vi "Central Update.vi"(11 "ref in":refnum<k20>) -> (3 "ref out":refnum<k20>)   [LabVIEW 2019]
uses:
  RT Controls/Top Dome Status.ctl
  RT Controls/FPGA State.ctl
  RT Controls/Main Box Status.ctl
  RT Controls/Rotation Status.ctl
  RT Controls/Last Rotation.ctl
  RT Controls/Homing State.ctl
  RT Controls/Main Box Config.ctl
  RT Controls/Main Box Control.ctl
  RT Controls/Main Box Buttons.ctl
  <vilib>/Utility/error.llb/Error Cluster From Error Code.vi
  <vilib>/rvi/errors/niLvFpgaAdjustHostInterfaceError.vi
  <vilib>/rvi/interface/nirviReadWriteControl/nirviReadWriteControl.xnode
  <vilib>/rvi/interface/Simulation/niFpgaSimulationCallBeginRW.vi
  NiFpgaLv.dll
panel:
  out "shutdown":bool
  out "FPGA State":T1
  out "mode":u8
  out "sub mode":u8
  out "cmd":i8
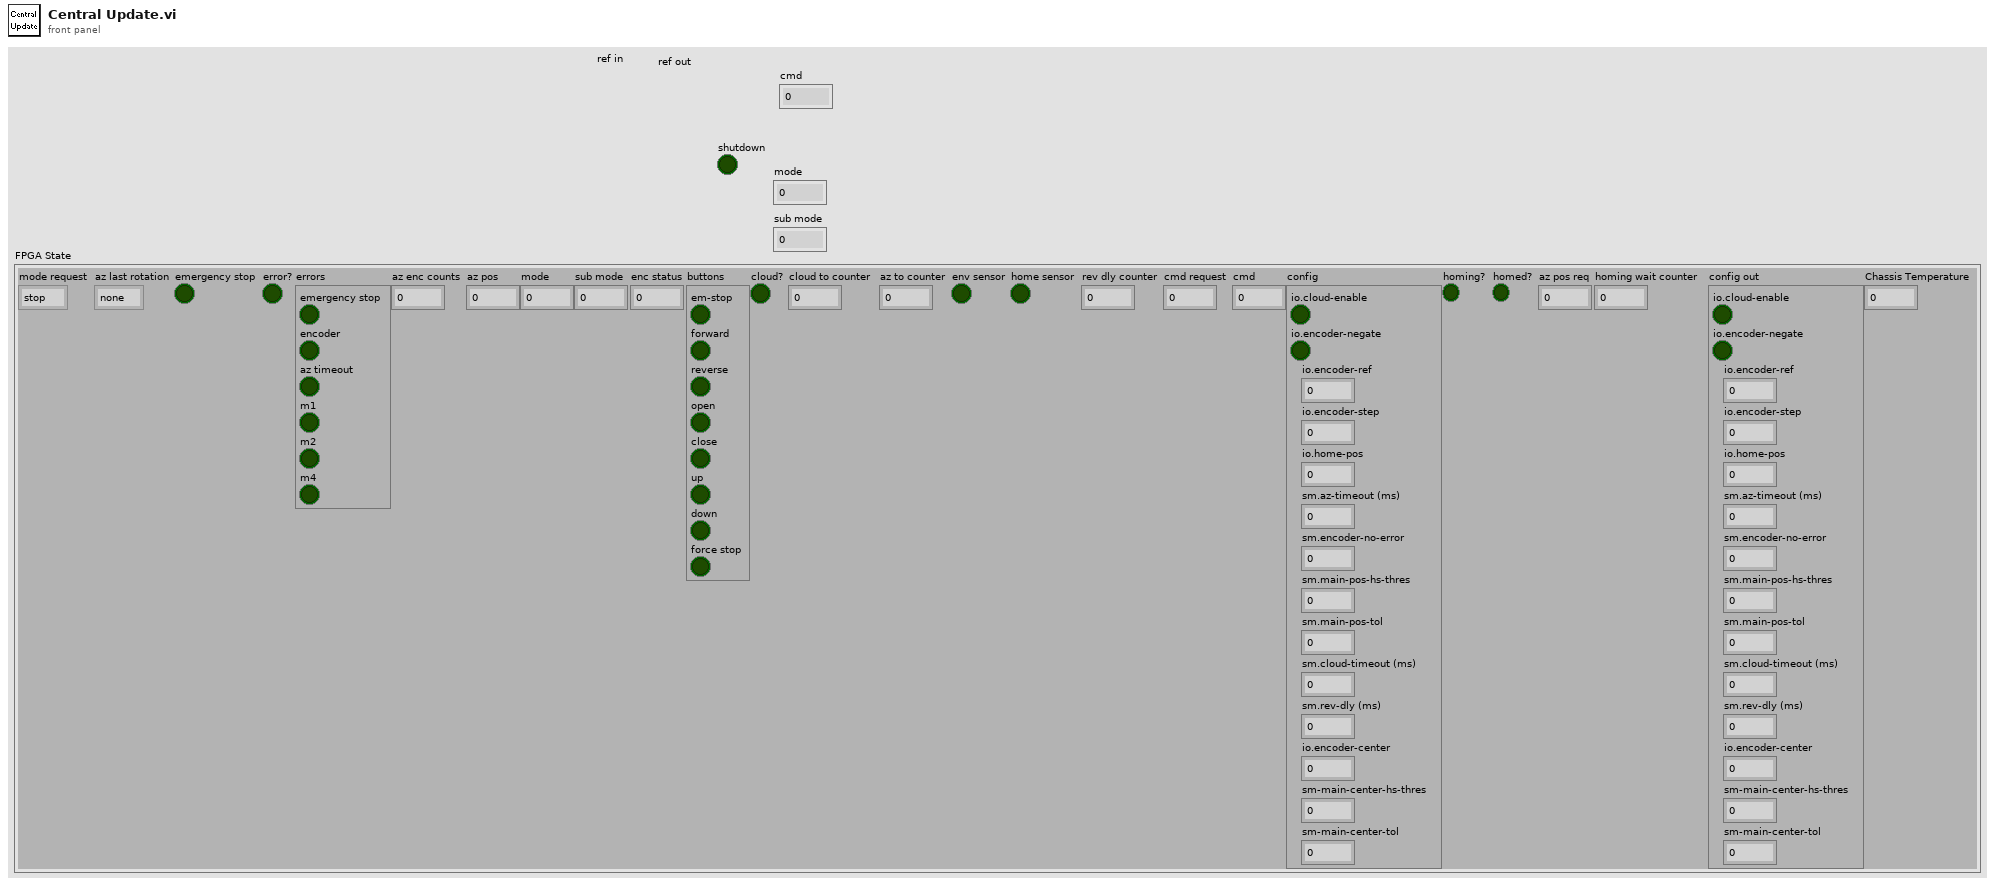
[diagram p1: front panel]
types:
  T1 = cluster{"mode request":enum16{"stop", "home", "position", "center"}, "az last rotation":enum16{"none", "forward", "reverse"}, "emergency stop":bool, "error?":bool, "errors":cluster{"emergency stop":bool, "encoder":bool, "az timeout":bool, "m1":bool, "m2":bool, "m4":bool}, "az enc counts":u64, "az pos":fxp<+/-,32,2>, "mode":u8, "sub mode":u8, "enc status":u16, "buttons":cluster{"em-stop":bool, "forward":bool, "reverse":bool, "open":bool, "close":bool, "up":bool, "down":bool, "force stop":bool}, "cloud?":bool, "cloud to counter":u32, "az to counter":u32, "env sensor":bool, "home sensor":bool, "rev dly counter":u32, "cmd request":i8, "cmd":i8, "config":cluster{"io.cloud-enable":bool, "io.encoder-negate":bool, "io.encoder-ref":u64, "io.encoder-step":u64, "io.home-pos":fxp<+/-,32,2>, "sm.az-timeout (ms)":u32, "sm.encoder-no-error":u16, "sm.main-pos-hs-thres":fxp<+/-,32,2>, "sm.main-pos-tol":fxp<+/-,32,2>, "sm.cloud-timeout (ms)":u32, "sm.rev-dly (ms)":u32, "io.encoder-center":u64, "sm-main-center-hs-thres":u64, "sm-main-center-tol":u64}, "homing?":bool, "homed?":bool, "az pos req":fxp<+/-,32,2>, "homing wait counter":u32, "config out":cluster{"io.cloud-enable":bool, "io.encoder-negate":bool, "io.encoder-ref":u64, "io.encoder-step":u64, "io.home-pos":fxp<+/-,32,2>, "sm.az-timeout (ms)":u32, "sm.encoder-no-error":u16, "sm.main-pos-hs-thres":fxp<+/-,32,2>, "sm.main-pos-tol":fxp<+/-,32,2>, "sm.cloud-timeout (ms)":u32, "sm.rev-dly (ms)":u32, "io.encoder-center":u64, "sm-main-center-hs-thres":u64, "sm-main-center-tol":u64}, "Chassis Temperature":i16}
  T2 = typedef "Homing State.ctl" = enum16{"Idle", "SlewFwd", "SlewRev", "SeekFwd", "SeekRev", "AtHome", "FwdWait", "RevWait"}
  T3 = typedef "Last Rotation.ctl" = enum16{"--", "RR", "RL"}
  T4 = typedef "Rotation Status.ctl" = enum16{"Stop", "Left", "Right", "Homing"}
  T5 = typedef "Top Dome Status.ctl" = cluster{"UpperDoorStatus":enum16{"Ajar", "Open", "Shut", "Error"}, "LowerDoorStatus":enum16{"Ajar", "Shut", "Open", "Error"}, "EM Button":bool, "WDTime":bool, "AutoShut":bool, "Rain":bool, "Interlock":bool, "UpperDoorEl":dbl, "LowerDoorEl":dbl, "UpperDoorEnc":u64, "LowerDoorEnc":u64}
  T6 = cluster{"emergency stop":bool, "encoder":bool, "az timeout":bool, "m1":bool, "m2":bool, "m4":bool}
  T7 = cluster{"em-stop":bool, "forward":bool, "reverse":bool, "open":bool, "close":bool, "up":bool, "down":bool, "force stop":bool}
  T8 = cluster{"io.cloud-enable":bool, "io.encoder-negate":bool, "io.encoder-ref":u64, "io.encoder-step":u64, "io.home-pos":fxp<+/-,32,2>, "sm.az-timeout (ms)":u32, "sm.encoder-no-error":u16, "sm.main-pos-hs-thres":fxp<+/-,32,2>, "sm.main-pos-tol":fxp<+/-,32,2>, "sm.cloud-timeout (ms)":u32, "sm.rev-dly (ms)":u32, "io.encoder-center":u64, "sm-main-center-hs-thres":u64, "sm-main-center-tol":u64}
  T9 = typedef "Main Box Config.ctl" = cluster{"WatchdogTim":i32, "DirRevDel":i32, "Coast":dbl, "HSThres":dbl, "EncCounts360":u64, "HomePos":dbl, "EncRefDeg":dbl, "EncRefCounts":u64, "Tol":dbl, "CloudEn":bool, "AutoShutEn":bool, "RainTim":i32, "AZTimeout":i32, "AZEncPol":enum16{"Positive", "Negative"}}
  T10 = typedef "Main Box Status.ctl" = cluster{"RotStatus":T4, "EMButton":bool, "TopComms":bool, "CurAZ":dbl, "At Home":bool, "LastRot":T3, "Cloud":bool, "CurAZEnc":u64, "LastAZ":dbl, "AutoShut":bool, "WDTime":bool, "HomeState":T2}
  T11 = typedef "Main Box Control.ctl" = cluster{"ForwardDome":bool, "ReverseDome":bool, "GotoHome":bool, "HighSpeed":bool}
  T12 = typedef "Main Box Buttons.ctl" = cluster{"EMStop":bool, "CloseMainDoor":bool, "OpenMainDoor":bool, "CloseLowerDoor":bool, "OpenLowerDoor":bool, "ForwardDome":bool, "ReverseDome":bool}
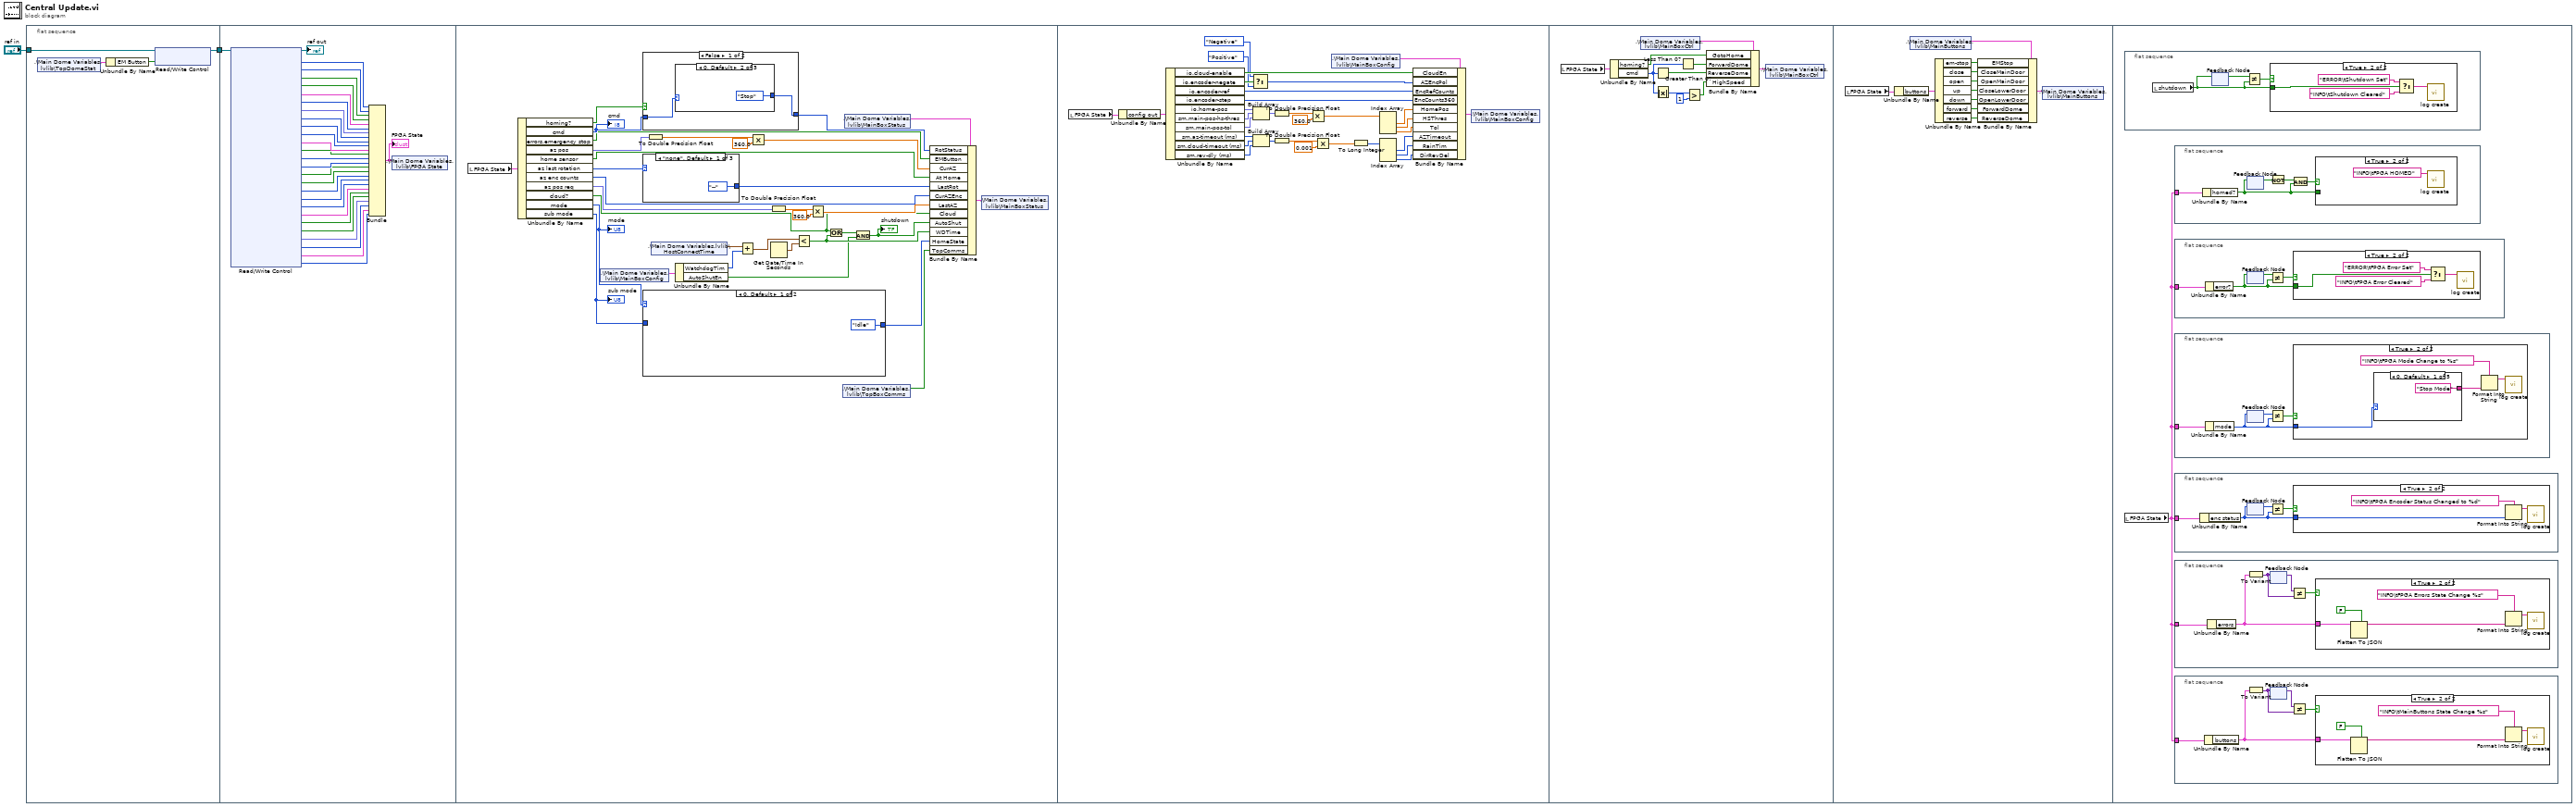
[diagram p0: block diagram]
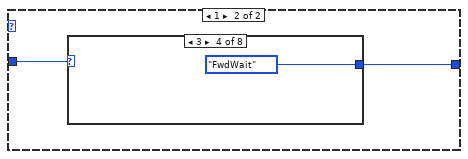
[diagram p2: hidden frame]
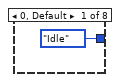
[diagram p3: hidden frame]
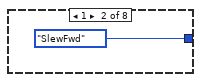
[diagram p4: hidden frame]
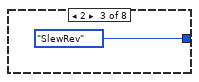
[diagram p5: hidden frame]
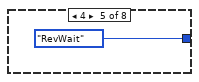
[diagram p6: hidden frame]
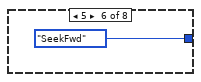
[diagram p7: hidden frame]
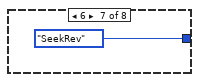
[diagram p8: hidden frame]
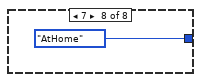
[diagram p9: hidden frame]
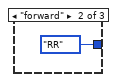
[diagram p10: hidden frame]
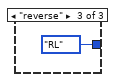
[diagram p11: hidden frame]
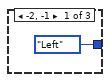
[diagram p12: hidden frame]
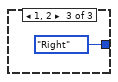
[diagram p13: hidden frame]
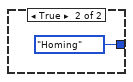
[diagram p14: hidden frame]
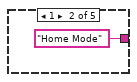
[diagram p20: hidden frame]
diagram:
  n1 = flat-sequence {
    tunnel: "ref in" -> [w6]
    tunnel: [w5] -> w2
    tunnel: w2 -> [w35]
    frame #0 {
      n2 = shared-variable ".\\Main Dome Variables.lvlib\\TopDomeStat"() -> (w4:T5)  [unwired: 1 in, 1 out]
      n3 = Unbundle By Name(w4) -> ("EM Button"=w3:bool)
      n4 = xnode "Read/Write Control"("FPGA VI Reference In"=w6, "emergency stop"=w3) -> ("FPGA VI Reference Out"=w5:refnum<k20>)  [unwired: 1 in, 1 out]
    }
    frame #1 {
      n5 = xnode "Read/Write Control"("FPGA VI Reference In"=w35) -> ("FPGA VI Reference Out"=→"ref out":refnum<k20>, "mode request"=w34:enum16{"stop", "home", "position", "center"}, "az last rotation"=w33:enum16{"none", "forward", "reverse"}, "emergency stop"=w32:bool, "error?"=w31:bool, "errors"=w30:T6, "az enc counts"=w29:u64, "az pos"=w28:fxp<+/-,32,2>, "mode"=w27:u8, "sub mode"=w26:u8, "enc status"=w25:u16, "buttons"=w24:T7, "cloud?"=w23:bool, "cloud to counter"=w22:u32, "az to counter"=w21:u32, "env sensor"=w20:bool, "home sensor"=w19:bool, "rev dly counter"=w18:u32, "cmd request"=w17:i8, "cmd"=w16:i8, "config"=w15:T8, "homing?"=w14:bool, "homed?"=w9:bool, "az pos req"=w13:fxp<+/-,32,2>, "homing wait counter"=w12:u32, "config out"=w11:T8, "Chassis Temperature"=w10:i16)  [unwired: 1 in, 1 out]
      n6 = Bundle("mode request"=w34, "az last rotation"=w33, "emergency stop"=w32, "error?"=w31, "errors"=w30, "az enc counts"=w29, "az pos"=w28, "mode"=w27, "sub mode"=w26, "enc status"=w25, "buttons"=w24, "cloud?"=w23, "cloud to counter"=w22, "az to counter"=w21, "env sensor"=w20, "home sensor"=w19, "rev dly counter"=w18, "cmd request"=w17, "cmd"=w16, "config"=w15, "homing?"=w14, "homed?"=w9, "az pos req"=w13, "homing wait counter"=w12, "config out"=w11, "Chassis Temperature"=w10) -> (w7:T1)  [unwired: 1 in]
      "FPGA State" <- w7
      n7 = shared-variable ".\\Main Dome Variables.lvlib\\FPGA State"(w7) -> ()  [unwired: 1 in, 1 out]
    }
    frame #2 {
      n8 = local read "FPGA State"() -> (w53:T1)
      n9 = Unbundle By Name(w53) -> ("homing?"=w52:bool, "cmd"=w51:i8, "errors.emergency stop"=w44:bool, "az pos"=w50:fxp<+/-,32,2>, "home sensor"=w43:bool, "az last rotation"=w49:enum16{"none", "forward", "reverse"}, "az enc counts"=w48:u64, "az pos req"=w47:fxp<+/-,32,2>, "cloud?"=w36:bool, "mode"=w46:u8, "sub mode"=w45:u8)
      "cmd" <- w51
      "sub mode" <- w45
      "mode" <- w46
      n10 = shared-variable ".\\Main Dome Variables.lvlib\\MainBoxConfig"() -> (w66:T9)  [unwired: 1 in, 1 out]
      n11 = case shown="False" w52 {
        tunnel: [w83 Rotation_Status."Homing" ("RotStatus")] -> w55
        tunnel: w51 -> [w84 _]
        frame False {
          n12 = case shown="0, Default" w84 {
            tunnel: [Rotation_Status."Left" ("RotStatus") Rotation_Status."Stop" ("RotStatus") Rotation_Status."Right" ("RotStatus")] -> w83
            frame -2, -1 {
            }
            frame 0, Default {
            }
            frame 1, 2 {
            }
          }
        }
        frame True {
        }
      }
      n13 = case shown="\"none\", Default" w49 {
        tunnel: [Last_Rotation."--" ("LastRot") Last_Rotation."RR" ("LastRot") Last_Rotation."RL" ("LastRot")] -> w59
        frame "none", Default {
        }
        frame "forward" {
        }
        frame "reverse" {
        }
      }
      n14 = case shown="0, Default" w46 {
        tunnel: [Homing_State."Idle" ("HomeState") w70] -> w37
        tunnel: w45 -> [_ w71]
        frame 0, Default {
        }
        frame 1 {
          n15 = case shown="3" w71 {
            tunnel: [Homing_State."Idle" ("HomeState") Homing_State."SlewFwd" ("HomeState") Homing_State."SlewRev" ("HomeState") Homing_State."FwdWait" ("HomeState") Homing_State."RevWait" ("HomeState") Homing_State."SeekFwd" ("HomeState") Homing_State."SeekRev" ("HomeState") Homing_State."AtHome" ("HomeState")] -> w70
            frame 0, Default {
            }
            frame 1 {
            }
            frame 2 {
            }
            frame 3 {
            }
            frame 4 {
            }
            frame 5 {
            }
            frame 6 {
            }
            frame 7 {
            }
          }
        }
      }
      n16 = To Double Precision Float(number=w50) -> (double precision float=w56:dbl)
      n17 = shared-variable ".\\Main Dome Variables.lvlib\\HostConnectTime"() -> (w42:timestamp)  [unwired: 1 in, 1 out]
      n18 = Unbundle By Name(w66) -> ("WatchdogTim"=w67:i32, "AutoShutEn"=w38:bool)
      n19 = Add(x=w42, y=w67) -> (x+y=w68:timestamp)
      n20 = Multiply(x=w56, y=360.0) -> (x*y=w58:dbl)
      n21 = To Double Precision Float(number=w47) -> (double precision float=w61:dbl)
      n22 = Get Date/Time In Seconds() -> (seconds since 1Jan1904=w64:timestamp)
      n23 = Less?(x=w68, y=w64) -> (x < y?=w40:bool)
      n24 = Multiply(x=w61, y=360.0) -> (x*y=w62:dbl)
      n25 = Or(x=w36, y=w40) -> (x .or. y?=w39:bool)
      n26 = shared-variable ".\\Main Dome Variables.lvlib\\TopBoxComms"() -> (w65:bool)  [unwired: 1 in, 1 out]
      n27 = shared-variable ".\\Main Dome Variables.lvlib\\MainBoxStatus"() -> (w54:T10)  [unwired: 1 in, 1 out]
      n28 = And(x=w39, y=w38) -> (x .and. y?=w41:bool)
      "shutdown" <- w41
      n29 = Bundle By Name(cluster=w54, "RotStatus"=w55, "EMButton"=w44, "CurAZ"=w58, "At Home"=w43, "LastRot"=w59, "CurAZEnc"=w48, "LastAZ"=w62, "Cloud"=w36, "AutoShut"=w41, "WDTime"=w40, "HomeState"=w37, "TopComms"=w65) -> (w63:T10)
      n30 = shared-variable ".\\Main Dome Variables.lvlib\\MainBoxStatus"(w63) -> ()  [unwired: 1 in, 1 out]
    }
    frame #3 {
      n31 = local read "FPGA State"() -> (w90:T1)
      n32 = Unbundle By Name(w90) -> ("config out"=w89:T8)
      n33 = Unbundle By Name(w89) -> ("io.cloud-enable"=w113:bool, "io.encoder-negate"=w112:bool, "io.encoder-ref"=w107:u64, "io.encoder-step"=w106:u64, "io.home-pos"=w120:fxp<+/-,32,2>, "sm.main-pos-hs-thres"=w119:fxp<+/-,32,2>, "sm.main-pos-tol"=w118:fxp<+/-,32,2>, "sm.az-timeout (ms)"=w117:u32, "sm.cloud-timeout (ms)"=w116:u32, "sm.rev-dly (ms)"=w115:u32)
      n34 = Select(t=enum16{"Positive", "Negative"}."Negative", s=w112, f=enum16{"Positive", "Negative"}."Positive" ("AZEncPol")) -> (s? t:f=w109:enum16{"Positive", "Negative"})
      n35 = Build Array(w120, w119, w118) -> (w96:fxp<+/-,32,2>[])
      n36 = Build Array(w117, w116, w115) -> (w94:u32[])
      n37 = To Double Precision Float(number=w96) -> (double precision float=w95:dbl[])
      n38 = To Double Precision Float(number=w94) -> (double precision float=w93:dbl[])
      n39 = Multiply(x=w95, y=360.0) -> (x*y=w105:dbl[])
      n40 = Multiply(x=w93, y=0.001) -> (x*y=w101:dbl[])
      n41 = shared-variable ".\\Main Dome Variables.lvlib\\MainBoxConfig"() -> (w114:T9)  [unwired: 1 in, 1 out]
      n42 = To Long Integer(number=w101) -> (32bit integer=w100:i32[])
      n43 = Index Array(array=w105) -> (element #1=w104:dbl, element #2=w103:dbl, element #3=w102:dbl)  [unwired: 3 in]
      n44 = Index Array(array=w100) -> (element #1=w99:i32, element #2=w98:i32, element #3=w97:i32)  [unwired: 3 in]
      n45 = Bundle By Name(cluster=w114, "CloudEn"=w113, "AZEncPol"=w109, "EncRefCounts"=w107, "EncCounts360"=w106, "HomePos"=w104, "HSThres"=w103, "Tol"=w102, "AZTimeout"=w99, "RainTim"=w98, "DirRevDel"=w97) -> (w108:T9)
      n46 = shared-variable ".\\Main Dome Variables.lvlib\\MainBoxConfig"(w108) -> ()  [unwired: 1 in, 1 out]
    }
    frame #4 {
      n47 = local read "FPGA State"() -> (w123:T1)
      n48 = Unbundle By Name(w123) -> ("homing?"=w122:bool, "cmd"=w121:i8)
      n49 = shared-variable ".\\Main Dome Variables.lvlib\\MainBoxCtrl"() -> (w130:T11)  [unwired: 1 in, 1 out]
      n50 = Less Than 0?(x=w121) -> (x < 0?=w125:bool)
      n51 = Absolute Value(x=w121) -> (abs(x)=w128:i8)
      n52 = Greater Than 0?(x=w121) -> (x > 0?=w124:bool)
      n53 = Greater?(x=w128, y=i8 1) -> (0:w126:bool)
      n54 = Bundle By Name(cluster=w130, "GotoHome"=w122, "ForwardDome"=w124, "ReverseDome"=w125, "HighSpeed"=w126) -> (w129:T11)
      n55 = shared-variable ".\\Main Dome Variables.lvlib\\MainBoxCtrl"(w129) -> ()  [unwired: 1 in, 1 out]
    }
    frame #5 {
      n56 = local read "FPGA State"() -> (w132:T1)
      n57 = Unbundle By Name(w132) -> ("buttons"=w131:T7)
      n58 = shared-variable ".\\Main Dome Variables.lvlib\\MainButtons"() -> (w141:T12)  [unwired: 1 in, 1 out]
      n59 = Unbundle By Name(w131) -> ("em-stop"=w140:bool, "close"=w139:bool, "open"=w138:bool, "up"=w135:bool, "down"=w134:bool, "forward"=w136:bool, "reverse"=w137:bool)
      n60 = Bundle By Name(cluster=w141, "EMStop"=w140, "CloseMainDoor"=w139, "OpenMainDoor"=w138, "CloseLowerDoor"=w135, "OpenLowerDoor"=w134, "ForwardDome"=w136, "ReverseDome"=w137) -> (w133:T12)
      n61 = shared-variable ".\\Main Dome Variables.lvlib\\MainButtons"(w133) -> ()  [unwired: 1 in, 1 out]
    }
    frame #6 {
      n62 = flat-sequence {
        frame #0 {
          n63 = local read "shutdown"() -> (w144:bool)
          n64 = feedback #1() -> (w143:bool)  [unwired: 1 in]
          n65 = feedback-in #1(w144) -> ()
          n66 = Not Equal?(x=w143, y=w144) -> (x != y?=w145:bool)
          n67 = case shown="True" w145 {
            tunnel: w144 -> [_ w146]
            frame False {
            }
            frame True {
              n68 = Select(t="ERROR\tShutdown Set" ("message"), s=w146, f="INFO\tShutdown Cleared" ("message")) -> (s? t:f=w147:string)
              n69 = call "log create.vi"("message"=w147) -> ()  [unwired: 11 in]
            }
          }
        }
      }
      n70 = local read "FPGA State"() -> (w142:T1)
      n71 = flat-sequence {
        tunnel: w142 -> [w154]
        frame #0 {
          n72 = Unbundle By Name(w154) -> ("homed?"=w153:bool)
          n73 = feedback #2() -> (w150:bool)  [unwired: 1 in]
          n74 = feedback-in #2(w153) -> ()
          n75 = Not(x=w150) -> (.not. x?=w151:bool)
          n76 = And(x=w151, y=w153) -> (x .and. y?=w152:bool)
          n77 = case shown="True" w152 {
            tunnel: w153 -> [_ _]
            frame False {
            }
            frame True {
              n78 = call "log create.vi"("message"="INFO\tFPGA HOMED" ("format string")) -> ()  [unwired: 11 in]
            }
          }
        }
      }
      n79 = flat-sequence {
        tunnel: w142 -> [w187]
        frame #0 {
          n80 = Unbundle By Name(w187) -> ("error?"=w186:bool)
          n81 = feedback #3() -> (w189:bool)  [unwired: 1 in]
          n82 = feedback-in #3(w186) -> ()
          n83 = Not Equal?(x=w189, y=w186) -> (x != y?=w188:bool)
          n84 = case shown="True" w188 {
            tunnel: w186 -> [_ w190]
            frame False {
            }
            frame True {
              n85 = Select(t="ERROR\tFPGA Error Set" ("message"), s=w190, f="INFO\tFPGA Error Cleared" ("message")) -> (s? t:f=w191:string)
              n86 = call "log create.vi"("message"=w191) -> ()  [unwired: 11 in]
            }
          }
        }
      }
      n87 = flat-sequence {
        tunnel: w142 -> [w175]
        frame #0 {
          n88 = Unbundle By Name(w175) -> ("mode"=w173:u8)
          n89 = feedback #4() -> (w174:u8)  [unwired: 1 in]
          n90 = feedback-in #4(w173) -> ()
          n91 = Not Equal?(x=w174, y=w173) -> (x != y?=w176:bool)
          n92 = case shown="True" w176 {
            tunnel: w173 -> [_ w178]
            frame False {
            }
            frame True {
              n93 = case shown="0, Default" w178 {
                tunnel: ["Stop Mode" "Home Mode" "Position Mode" "Error Mode" "Center Mode"] -> w177
                frame 0, Default {
                }
                frame 1 {
                }
                frame 2 {
                }
                frame 3 {
                }
                frame 4 {
                }
              }
              n94 = Format Into String(format string="INFO\tFPGA Mode Change to %s", w177) -> (resulting string=w180:string)  [unwired: 2 in, 1 out]
              n95 = call "log create.vi"("message"=w180) -> ()  [unwired: 11 in]
            }
          }
        }
      }
      n96 = flat-sequence {
        tunnel: w142 -> [w168]
        frame #0 {
          n97 = Unbundle By Name(w168) -> ("enc status"=w166:u16)
          n98 = feedback #5() -> (w167:u16)  [unwired: 1 in]
          n99 = feedback-in #5(w166) -> ()
          n100 = Not Equal?(x=w167, y=w166) -> (x != y?=w169:bool)
          n101 = case shown="True" w169 {
            tunnel: w166 -> [_ w170]
            frame False {
            }
            frame True {
              n102 = Format Into String(format string="INFO\tFPGA Encoder Status Changed to %d", w170) -> (resulting string=w172:string)  [unwired: 2 in, 1 out]
              n103 = call "log create.vi"("message"=w172) -> ()  [unwired: 11 in]
            }
          }
        }
      }
      n104 = flat-sequence {
        tunnel: w142 -> [w160]
        frame #0 {
          n105 = Unbundle By Name(w160) -> ("errors"=w159:T6)
          n106 = To Variant(anything=w159) -> (Variant=w157:variant)
          n107 = feedback #6() -> (w158:variant)  [unwired: 1 in]
          n108 = feedback-in #6(w157) -> ()
          n109 = Not Equal?(x=w158, y=w157) -> (x != y?=w156:bool)
          n110 = case shown="True" w156 {
            tunnel: w159 -> [_ w161]
            frame False {
            }
            frame True {
              n111 = Flatten To JSON(enable LabVIEW extensions? (T)=FALSE, anything=w161) -> (JSON string=w162:string)  [unwired: 1 in, 1 out]
              n112 = Format Into String(format string="INFO\tFPGA Errors State Change %s", w162) -> (resulting string=w164:string)  [unwired: 2 in, 1 out]
              n113 = call "log create.vi"("message"=w164) -> ()  [unwired: 11 in]
            }
          }
        }
      }
      n114 = flat-sequence {
        tunnel: w142 -> [w198]
        frame #0 {
          n115 = Unbundle By Name(w198) -> ("buttons"=w196:T7)
          n116 = To Variant(anything=w196) -> (Variant=w195:variant)
          n117 = feedback #7() -> (w197:variant)  [unwired: 1 in]
          n118 = feedback-in #7(w195) -> ()
          n119 = Not Equal?(x=w197, y=w195) -> (x != y?=w194:bool)
          n120 = case shown="True" w194 {
            tunnel: w196 -> [_ w199]
            frame False {
            }
            frame True {
              n121 = Flatten To JSON(enable LabVIEW extensions? (T)=FALSE, anything=w199) -> (JSON string=w201:string)  [unwired: 1 in, 1 out]
              n122 = Format Into String(format string="INFO\tMainButtons State Change %s", w201) -> (resulting string=w203:string)  [unwired: 2 in, 1 out]
              n123 = call "log create.vi"("message"=w203) -> ()  [unwired: 11 in]
            }
          }
        }
      }
    }
  }
